vi "参数.vi"() -> ()   [LabVIEW 2018]
panel:
  in  "变频快速变化量":sgl caption="N" format="%.2f"
  in  "变频慢速变化量":sgl caption="N" format="%.2f"
  in  "变频变化周期":sgl caption="N" format="%.2f"
  in  "变频初始频率":sgl caption="N" format="%.2f"
  out "信号":bool
  out "物料编号":string
  out "机台编号":string
  out "产线编号":string
  in  "选项卡控件":enum32{"出风口", "信号显示"}(tab)
  in  "1#选项卡控件":enum32{"拨钮左到右", "拨钮右到左", "拨钮下到上", "拨钮上到下"}(tab)
  in  "1#拨钮左右-系数+":sgl=10.0 caption="操作力系数+" format="%.2f"
  in  "1#拨钮左右-基准":sgl=10.0 caption="操作力基准" format="%.2f"
  in  "1#拨钮左右-上参考":sgl=10.0 caption="操作力上参考" format="%.2f"
  in  "1#拨钮左右-下参考":sgl=10.0 caption="操作力下参考" format="%.2f"
  in  "1#拨钮左右-终点":dbl=10.0 caption="操作力终点" format="%.2f"
  in  "1#拨钮左右-起点":dbl=10.0 caption="操作力起点" format="%.2f"
  in  "1#拨钮左右-锁起点":dbl=10.0 caption="锁止力起点" format="%.2f"
  in  "1#拨钮左右-锁终点":dbl=10.0 caption="锁止力终点" format="%.2f"
  in  "1#拨钮左右-锁系数+":sgl=10.0 caption="锁止力系数+" format="%.2f"
  in  "1#拨钮左右-锁系数x":sgl=10.0 caption="锁止力系数x" format="%.2f"
  in  "1#拨钮左右-锁上限":sgl=10.0 caption="锁止力上限" format="%.2f"
  in  "1#拨钮左右-锁下限":sgl=10.0 caption="锁止力下限" format="%.2f"
  in  "1#拨钮左右-系数x":sgl=10.0 caption="操作力系数x" format="%.2f"
  in  "1#拨钮左右-曲线点数":dbl=10.0 caption="曲线点数"
  in  "1#拨钮左右-上限":sgl=10.0 caption="操作力上限" format="%.2f"
  in  "1#拨钮左右-下限":sgl=10.0 caption="操作力下限" format="%.2f"
  in  "1#拨钮左右-Y轴上限":dbl=10.0 caption="Y轴上限" format="%.1f"
  in  "1#拨钮左右-Y轴下限":dbl=10.0 caption="Y轴下限" format="%.1f"
  in  "1#拨钮右左-系数+":sgl=10.0 caption="操作力系数+" format="%.2f"
  in  "1#拨钮右左-基准":sgl=10.0 caption="操作力基准" format="%.2f"
  in  "1#拨钮右左上参考":sgl=10.0 caption="操作力上参考" format="%.2f"
  in  "1#拨钮右左-下参考":sgl=10.0 caption="操作力下参考" format="%.2f"
  in  "1#拨钮右左-终点":dbl=10.0 caption="操作力终点" format="%.2f"
  in  "1#拨钮右左-起点":dbl=10.0 caption="操作力起点" format="%.2f"
  in  "1#拨钮右左-锁起点":dbl=10.0 caption="锁止力起点" format="%.2f"
  in  "1#拨钮右左-锁终点":dbl=10.0 caption="锁止力终点" format="%.2f"
  in  "1#拨钮右左-锁系数+":sgl=10.0 caption="锁止力系数+" format="%.2f"
  in  "1#拨钮右左-锁系数x":sgl=10.0 caption="锁止力系数x" format="%.2f"
  in  "1#拨钮右左-锁上限":sgl=10.0 caption="锁止力上限" format="%.2f"
  in  "1#拨钮右左-锁下限":sgl=10.0 caption="锁止力下限" format="%.2f"
  in  "1#拨钮右左-系数x":sgl=10.0 caption="操作力系数x" format="%.2f"
  in  "1#拨钮右左-曲线点数":dbl=10.0 caption="曲线点数"
  in  "1#拨钮右左-上限":sgl=10.0 caption="操作力上限" format="%.2f"
  in  "1#拨钮右左-下限":sgl=10.0 caption="操作力下限" format="%.2f"
  in  "1#拨钮右左-Y轴上限":dbl=10.0 caption="Y轴上限" format="%.1f"
  in  "1#拨钮右左-Y轴下限":dbl=10.0 caption="Y轴下限" format="%.1f"
  in  "1#拨钮下上-系数+":sgl=10.0 caption="操作力系数+" format="%.2f"
  in  "1#拨钮下上-基准":sgl=10.0 caption="操作力基准" format="%.2f"
  in  "1#拨钮下上-上参考":sgl=10.0 caption="操作力上参考" format="%.2f"
  in  "1#拨钮下上-下参考":sgl=10.0 caption="操作力下参考" format="%.2f"
  in  "1#拨钮下上-终点":dbl=10.0 caption="操作力终点" format="%.2f"
  in  "1#拨钮下上-起点":dbl=10.0 caption="操作力起点" format="%.2f"
  in  "1#拨钮下上-系数x":sgl=10.0 caption="操作力系数x" format="%.2f"
  in  "1#拨钮下上-曲线点数":dbl=10.0 caption="曲线点数"
  in  "1#拨钮下上-上限":sgl=10.0 caption="操作力上限" format="%.2f"
  in  "1#拨钮下上-下限":sgl=10.0 caption="操作力下限" format="%.2f"
  in  "1#拨钮下上-Y轴上限":dbl=10.0 caption="Y轴上限" format="%.1f"
  in  "1#拨钮下上-Y轴下限":dbl=10.0 caption="Y轴下限" format="%.1f"
  in  "1#拨钮上下-系数+":sgl=10.0 caption="操作力系数+" format="%.2f"
  in  "1#拨钮上下-基准":sgl=10.0 caption="操作力基准" format="%.2f"
  in  "1#拨钮上下-上参考":sgl=10.0 caption="操作力上参考" format="%.2f"
  in  "1#拨钮上下-下参考":sgl=10.0 caption="操作力下参考" format="%.2f"
  in  "1#拨钮上下-终点":dbl=10.0 caption="操作力终点" format="%.2f"
  in  "1#拨钮上下-起点":dbl=10.0 caption="操作力起点" format="%.2f"
  in  "1#拨钮上下-系数x":sgl=10.0 caption="操作力系数x" format="%.2f"
  in  "1#拨钮上下-曲线点数":dbl=10.0 caption="曲线点数"
  in  "1#拨钮上下-上限":sgl=10.0 caption="操作力上限" format="%.2f"
  in  "1#拨钮上下-下限":sgl=10.0 caption="操作力下限" format="%.2f"
  in  "1#拨钮上下-Y轴上限":dbl=10.0 caption="Y轴上限" format="%.1f"
  in  "1#拨钮上下-Y轴下限":dbl=10.0 caption="Y轴下限" format="%.1f"
  out "检测序号":u16 format="%05d"
  out "力":sgl[](array[numeric]) format="%.4f"
  out "PLC结果":T1
  out "检测步骤":T2
  out "PLC状态":T3
  in  "LOG":bool
  in  "伺服速度":sgl caption="N" format="%.1f"
  in  "气压稳定时间":sgl caption="N" format="%.1f"
  in  "LED电流下限":sgl caption="N" format="%.2f"
  in  "LED电流上限":sgl caption="N" format="%.2f"
  in  "风门开电压下限":sgl caption="N" format="%.2f"
  in  "风门开电压上限":sgl caption="N" format="%.2f"
  in  "风门闭电压下限":sgl caption="N" format="%.2f"
  in  "风门闭电压上限":sgl caption="N" format="%.2f"
  in  "压力下限":sgl caption="N" format="%.1f"
  in  "压力上限":sgl caption="N" format="%.1f"
  in  "泄漏量上限":sgl caption="N" format="%.2f"
  out "有值改变":bool
  in  "停止":bool
  in  "轮盘预压力":sgl caption="N" format="%.1f"
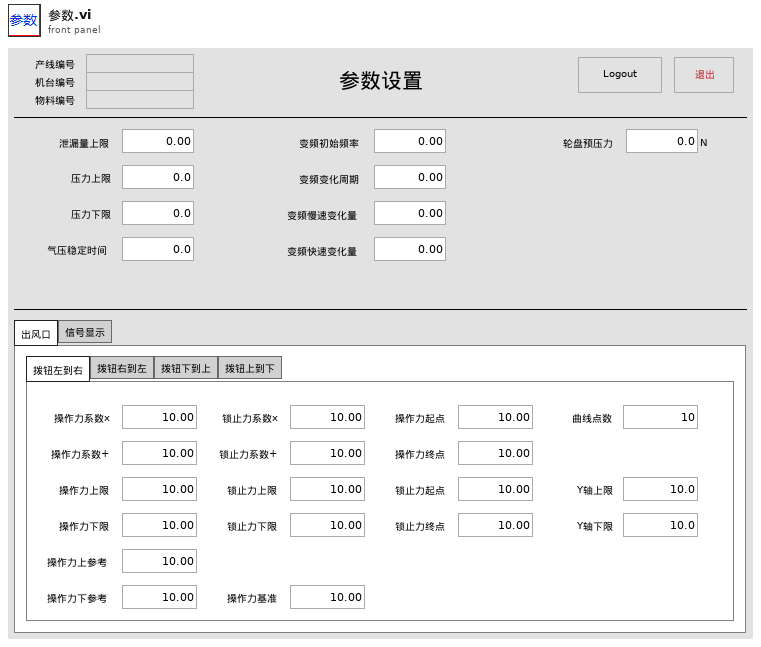
[diagram p1: front panel]
types:
  T1 = cluster{"1#泄漏量":bool, "1#风门闭电压":bool, "1#风门开电压":bool, "1#LED电压":bool, "1#LED电流":bool, "外观结果":bool, "2#泄漏量":bool, "2#风门闭电压":bool, "2#风门开电压":bool, "2#LED电压":bool, "2#LED电流":bool, "3#泄漏量":bool, "3#风门闭电压":bool, "3#风门开电压":bool, "3#LED电压":bool, "3#LED电流":bool}
  T2 = cluster{"泄漏量":bool, "风门开闭电检":bool, "LED电检":bool, "外观检测":bool, "1#轮盘关开":bool, "1#轮盘关开锁":bool, "1#轮盘开关":bool, "1#轮盘开关锁":bool, "1#拨钮左右":bool, "1#拨钮右左":bool, "1#拨钮上下":bool, "1#拨钮下上":bool, "2#轮盘关开":bool, "2#轮盘关开锁":bool, "2#轮盘开关":bool, "2#轮盘开关锁":bool, "2#拨钮左右":bool, "2#拨钮右左":bool, "2#拨钮上下":bool, "2#拨钮下上":bool, "3#轮盘关开":bool, "3#轮盘关开锁":bool, "3#轮盘开关":bool, "3#轮盘开关锁":bool, "3#拨钮左右":bool, "3#拨钮右左":bool, "3#拨钮上下":bool, "3#拨钮下上":bool}
  T3 = cluster{"PLC就绪":bool, "ROBOT就绪":bool, "空动作":bool, "检测NG":bool, "检测结束":bool, "检测开始":bool, "初始化脉冲":bool, "1#检测NG":bool, "2#检测NG":bool, "3#检测NG":bool}
  T4 = enum8{"Enabled", "Disabled", "Disabled and Grayed Out"}
  T5 = cluster{"轮盘预压力":sgl, "泄漏量上限":sgl, "压力上限":sgl, "压力下限":sgl, "风门闭电压上限":sgl, "风门闭电压下限":sgl, "风门开电压上限":sgl, "风门开电压下限":sgl, "LED电流上限":sgl, "LED电流下限":sgl, "气压稳定时间":sgl, "伺服速度":sgl, "INV初始频率":sgl, "INV变化周期":sgl, "INV慢速变化量":sgl, "INV快速变化量":sgl}
  T6 = cluster{"选择":enum16{"Fx", "Fy", "Fz", "Mx", "My", "Mz"}, "系数x":sgl, "系数+":sgl, "上限":sgl, "下限":sgl, "Ymax":dbl, "Ymin":dbl, "点数":dbl, "锁系数x":sgl, "锁上限":sgl, "锁下限":sgl, "锁系数+":sgl, "起点":dbl, "终点":dbl, "锁起点":dbl, "锁终点":dbl, "上参考":sgl, "下参考":sgl, "基准":sgl}
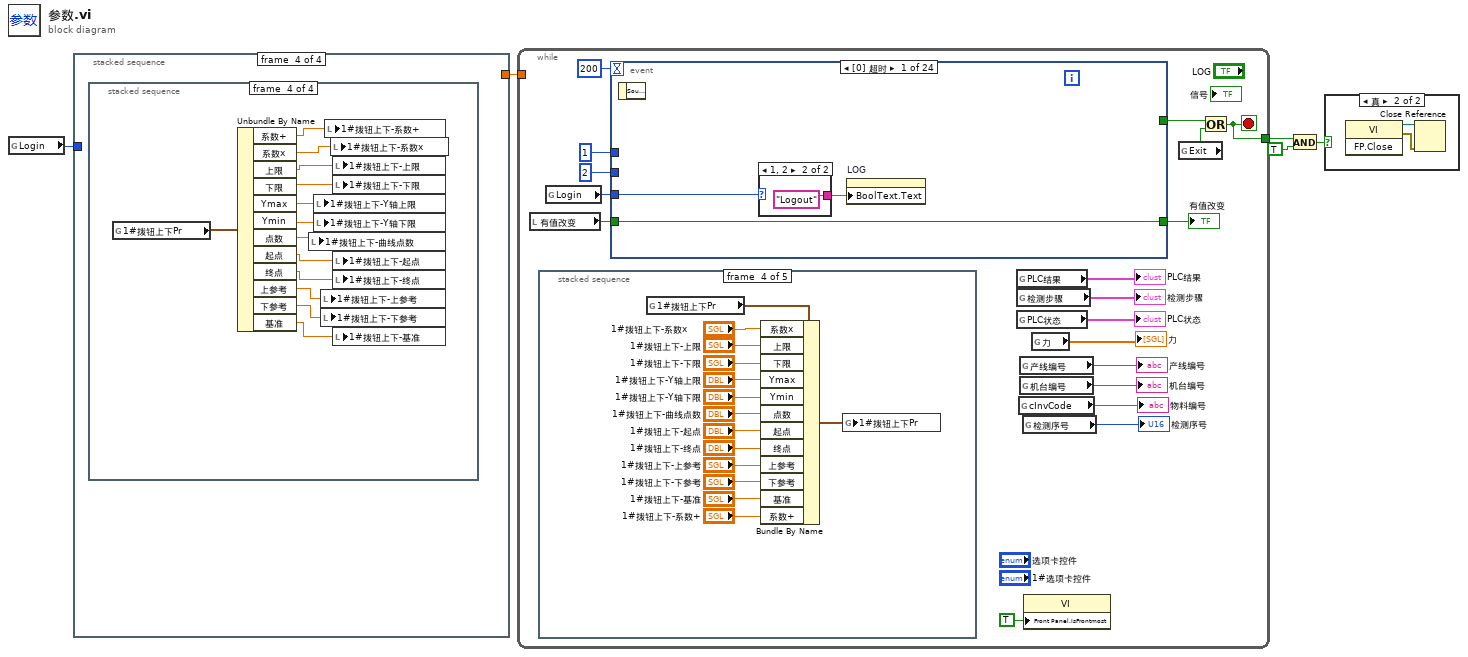
[diagram p0: block diagram]
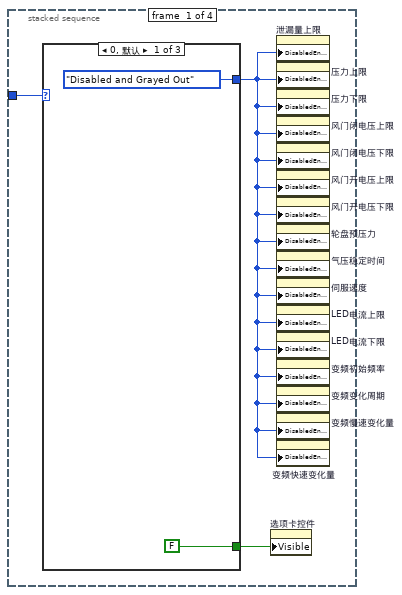
[diagram p2: hidden frame]
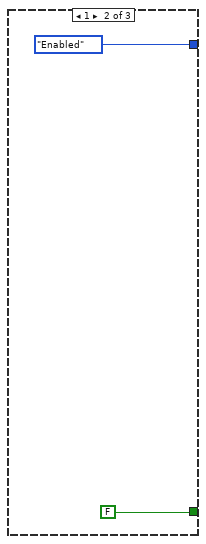
[diagram p3: hidden frame]
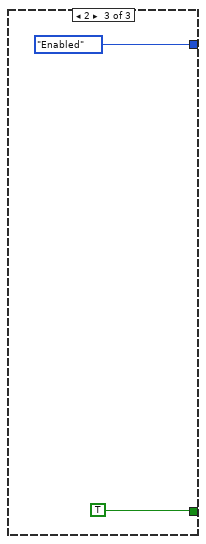
[diagram p4: hidden frame]
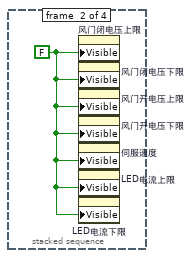
[diagram p5: hidden frame]
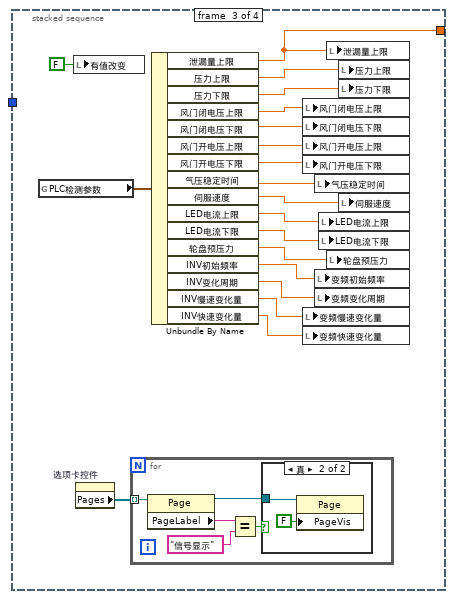
[diagram p6: hidden frame]
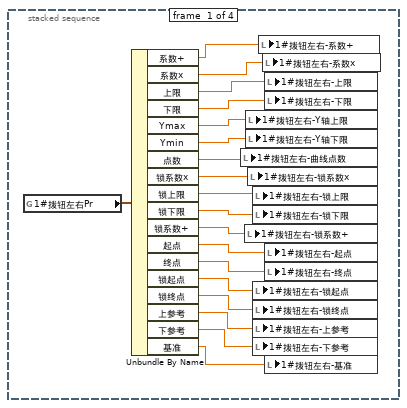
[diagram p8: hidden frame]
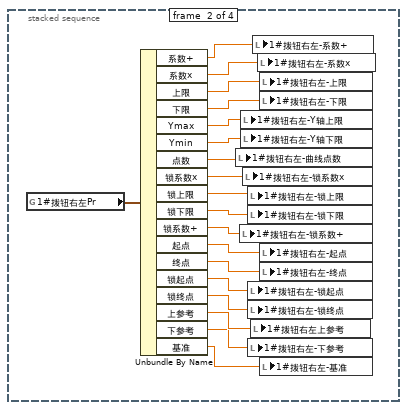
[diagram p9: hidden frame]
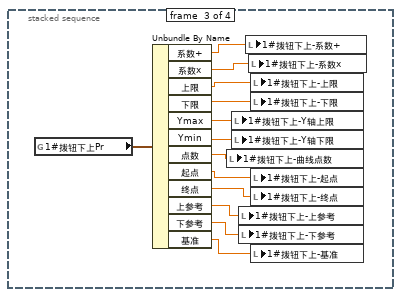
[diagram p10: hidden frame]
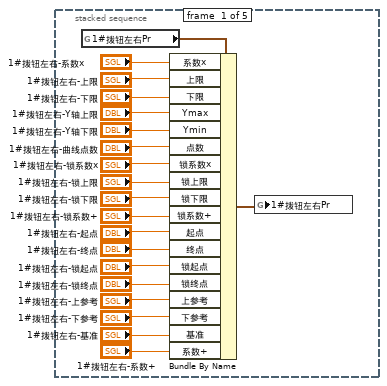
[diagram p12: hidden frame]
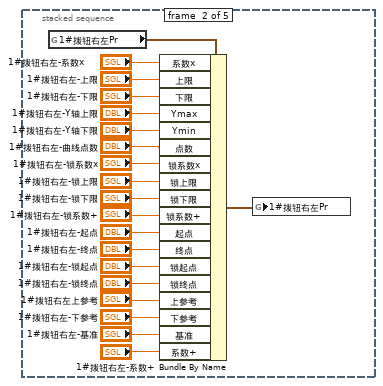
[diagram p13: hidden frame]
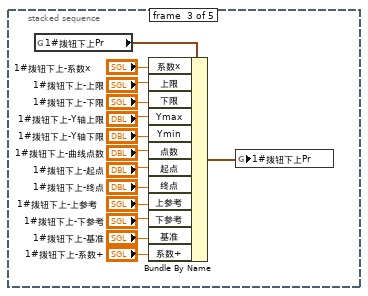
[diagram p14: hidden frame]
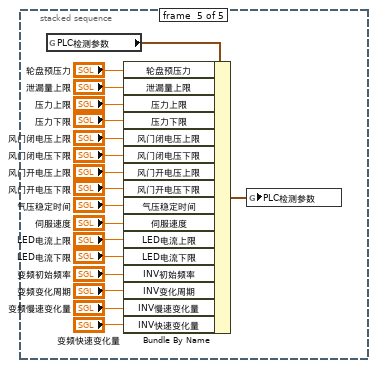
[diagram p15: hidden frame]
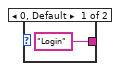
[diagram p16: hidden frame]
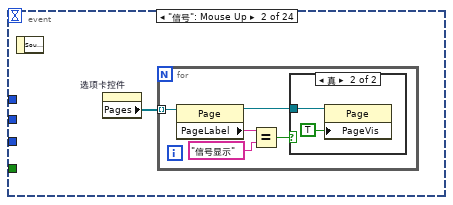
[diagram p17: hidden frame]
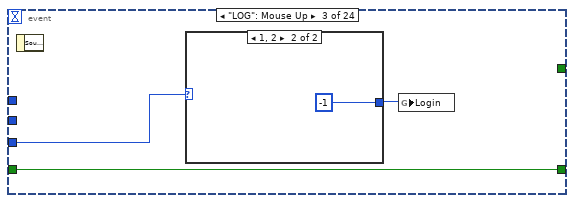
[diagram p19: hidden frame]
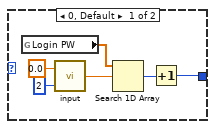
[diagram p20: hidden frame]
diagram:
  n1 = global read "全局 1.vi" "Login"() -> (w2:i32)
  n2 = stacked-sequence {
    tunnel: w2 -> [w8 _ _ _]
    tunnel: [_ _ w20 _] -> w1
    frame #0 {
      n3 = case shown="0, 默认" w8 {
        tunnel: [T4."Disabled and Grayed Out" ("禁用") T4."Enabled" ("禁用") T4."Enabled" ("禁用")] -> w6
        tunnel: [FALSE ("可见") FALSE ("可见") TRUE ("可见")] -> w7
        frame 0, Default {
        }
        frame 1 {
        }
        frame 2 {
        }
      }
      n4 = property on="选项卡控件" class="TabCtl (严格)"("Visible"=w7) -> ()  [unwired: 2 in, 2 out]
      n5 = property on="泄漏量上限" class="DigNum (严格)"("DisabledEnum"=w6) -> ()  [unwired: 2 in, 2 out]
      n6 = property on="压力上限" class="DigNum (严格)"("DisabledEnum"=w6) -> ()  [unwired: 2 in, 2 out]
      n7 = property on="压力下限" class="DigNum (严格)"("DisabledEnum"=w6) -> ()  [unwired: 2 in, 2 out]
      n8 = property on="风门闭电压上限" class="DigNum (严格)"("DisabledEnum"=w6) -> ()  [unwired: 2 in, 2 out]
      n9 = property on="风门闭电压下限" class="DigNum (严格)"("DisabledEnum"=w6) -> ()  [unwired: 2 in, 2 out]
      n10 = property on="风门开电压上限" class="DigNum (严格)"("DisabledEnum"=w6) -> ()  [unwired: 2 in, 2 out]
      n11 = property on="风门开电压下限" class="DigNum (严格)"("DisabledEnum"=w6) -> ()  [unwired: 2 in, 2 out]
      n12 = property on="轮盘预压力" class="DigNum (严格)"("DisabledEnum"=w6) -> ()  [unwired: 2 in, 2 out]
      n13 = property on="气压稳定时间" class="DigNum (严格)"("DisabledEnum"=w6) -> ()  [unwired: 2 in, 2 out]
      n14 = property on="伺服速度" class="DigNum (严格)"("DisabledEnum"=w6) -> ()  [unwired: 2 in, 2 out]
      n15 = property on="LED电流上限" class="DigNum (严格)"("DisabledEnum"=w6) -> ()  [unwired: 2 in, 2 out]
      n16 = property on="LED电流下限" class="DigNum (严格)"("DisabledEnum"=w6) -> ()  [unwired: 2 in, 2 out]
      n17 = property on="变频初始频率" class="DigNum (严格)"("DisabledEnum"=w6) -> ()  [unwired: 2 in, 2 out]
      n18 = property on="变频变化周期" class="DigNum (严格)"("DisabledEnum"=w6) -> ()  [unwired: 2 in, 2 out]
      n19 = property on="变频慢速变化量" class="DigNum (严格)"("DisabledEnum"=w6) -> ()  [unwired: 2 in, 2 out]
      n20 = property on="变频快速变化量" class="DigNum (严格)"("DisabledEnum"=w6) -> ()  [unwired: 2 in, 2 out]
    }
    frame #1 {
      w15 = FALSE ("可见")
      n21 = property on="风门闭电压上限" class="DigNum (严格)"("Visible"=w15) -> ()  [unwired: 2 in, 2 out]
      n22 = property on="风门闭电压下限" class="DigNum (严格)"("Visible"=w15) -> ()  [unwired: 2 in, 2 out]
      n23 = property on="风门开电压上限" class="DigNum (严格)"("Visible"=w15) -> ()  [unwired: 2 in, 2 out]
      n24 = property on="风门开电压下限" class="DigNum (严格)"("Visible"=w15) -> ()  [unwired: 2 in, 2 out]
      n25 = property on="伺服速度" class="DigNum (严格)"("Visible"=w15) -> ()  [unwired: 2 in, 2 out]
      n26 = property on="LED电流上限" class="DigNum (严格)"("Visible"=w15) -> ()  [unwired: 2 in, 2 out]
      n27 = property on="LED电流下限" class="DigNum (严格)"("Visible"=w15) -> ()  [unwired: 2 in, 2 out]
    }
    frame #2 {
      n28 = global read "全局 1.vi" "PLC检测参数"() -> (w24:T5)
      n29 = local write "有值改变"(FALSE ("有值改变")) -> ()
      n30 = property on="选项卡控件" class="TabCtl (严格)"() -> ("Pages"=w21:refnum<vi>[])  [unwired: 2 in, 2 out]
      n31 = for {
        tunnel: w21 -> [w36] mode=indexing
        n32 = property class="Page"(reference=w36) -> (reference out=w35:refnum<vi>, "PageLabel"=w39:string)  [unwired: 1 in, 1 out]
        n33 = Equal?(x=w39, y="信号显示") -> (x = y?=w37:bool)
        n34 = case shown="真" w37 {
          tunnel: w35 -> [_ w40]
          frame False {
          }
          frame True {
            n35 = property class="Page"(reference=w40, "PageVis"=FALSE ("选项卡可见")) -> ()  [unwired: 1 in, 2 out]
          }
        }
      }
      n36 = Unbundle By Name(w24) -> ("泄漏量上限"=w20:sgl, "压力上限"=w34:sgl, "压力下限"=w33:sgl, "风门闭电压上限"=w32:sgl, "风门闭电压下限"=w31:sgl, "风门开电压上限"=w30:sgl, "风门开电压下限"=w29:sgl, "气压稳定时间"=w28:sgl, "伺服速度"=w27:sgl, "LED电流上限"=w26:sgl, "LED电流下限"=w25:sgl, "轮盘预压力"=w22:sgl, "INV初始频率"=w16:sgl, "INV变化周期"=w17:sgl, "INV慢速变化量"=w18:sgl, "INV快速变化量"=w19:sgl)
      n37 = local write "风门闭电压上限"(w32) -> ()
      n38 = local write "风门闭电压下限"(w31) -> ()
      n39 = local write "风门开电压上限"(w30) -> ()
      n40 = local write "风门开电压下限"(w29) -> ()
      n41 = local write "变频慢速变化量"(w18) -> ()
      n42 = local write "变频快速变化量"(w19) -> ()
      n43 = local write "气压稳定时间"(w28) -> ()
      n44 = local write "变频初始频率"(w16) -> ()
      n45 = local write "变频变化周期"(w17) -> ()
      n46 = local write "LED电流上限"(w26) -> ()
      n47 = local write "LED电流下限"(w25) -> ()
      n48 = local write "泄漏量上限"(w20) -> ()
      n49 = local write "轮盘预压力"(w22) -> ()
      n50 = local write "压力上限"(w34) -> ()
      n51 = local write "压力下限"(w33) -> ()
      n52 = local write "伺服速度"(w27) -> ()
    }
    frame #3 {
      n53 = stacked-sequence {
        frame #0 {
          n54 = global read "全局F参数.vi" "1#拨钮左右Pr"() -> (w60:T6)
          n55 = Unbundle By Name(w60) -> ("系数+"=w42:sgl, "系数x"=w59:sgl, "上限"=w57:sgl, "下限"=w56:sgl, "Ymax"=w55:dbl, "Ymin"=w54:dbl, "点数"=w58:dbl, "锁系数x"=w51:sgl, "锁上限"=w53:sgl, "锁下限"=w52:sgl, "锁系数+"=w50:sgl, "起点"=w49:dbl, "终点"=w48:dbl, "锁起点"=w47:dbl, "锁终点"=w46:dbl, "上参考"=w45:sgl, "下参考"=w44:sgl, "基准"=w43:sgl)
          n56 = local write "1#拨钮左右-曲线点数"(w58) -> ()
          n57 = local write "1#拨钮左右-锁系数+"(w50) -> ()
          n58 = local write "1#拨钮左右-Y轴上限"(w55) -> ()
          n59 = local write "1#拨钮左右-Y轴下限"(w54) -> ()
          n60 = local write "1#拨钮左右-锁系数x"(w51) -> ()
          n61 = local write "1#拨钮左右-锁上限"(w53) -> ()
          n62 = local write "1#拨钮左右-锁下限"(w52) -> ()
          n63 = local write "1#拨钮左右-锁起点"(w47) -> ()
          n64 = local write "1#拨钮左右-锁终点"(w46) -> ()
          n65 = local write "1#拨钮左右-上参考"(w45) -> ()
          n66 = local write "1#拨钮左右-下参考"(w44) -> ()
          n67 = local write "1#拨钮左右-系数+"(w42) -> ()
          n68 = local write "1#拨钮左右-系数x"(w59) -> ()
          n69 = local write "1#拨钮左右-上限"(w57) -> ()
          n70 = local write "1#拨钮左右-下限"(w56) -> ()
          n71 = local write "1#拨钮左右-起点"(w49) -> ()
          n72 = local write "1#拨钮左右-终点"(w48) -> ()
          n73 = local write "1#拨钮左右-基准"(w43) -> ()
        }
        frame #1 {
          n74 = global read "全局F参数.vi" "1#拨钮右左Pr"() -> (w79:T6)
          n75 = Unbundle By Name(w79) -> ("系数+"=w61:sgl, "系数x"=w78:sgl, "上限"=w76:sgl, "下限"=w75:sgl, "Ymax"=w74:dbl, "Ymin"=w73:dbl, "点数"=w77:dbl, "锁系数x"=w72:sgl, "锁上限"=w71:sgl, "锁下限"=w70:sgl, "锁系数+"=w69:sgl, "起点"=w68:dbl, "终点"=w67:dbl, "锁起点"=w66:dbl, "锁终点"=w65:dbl, "上参考"=w64:sgl, "下参考"=w63:sgl, "基准"=w62:sgl)
          n76 = local write "1#拨钮右左-曲线点数"(w77) -> ()
          n77 = local write "1#拨钮右左-锁系数+"(w69) -> ()
          n78 = local write "1#拨钮右左-Y轴上限"(w74) -> ()
          n79 = local write "1#拨钮右左-Y轴下限"(w73) -> ()
          n80 = local write "1#拨钮右左-锁系数x"(w72) -> ()
          n81 = local write "1#拨钮右左-锁上限"(w71) -> ()
          n82 = local write "1#拨钮右左-锁下限"(w70) -> ()
          n83 = local write "1#拨钮右左-锁起点"(w66) -> ()
          n84 = local write "1#拨钮右左-锁终点"(w65) -> ()
          n85 = local write "1#拨钮右左-下参考"(w63) -> ()
          n86 = local write "1#拨钮右左上参考"(w64) -> ()
          n87 = local write "1#拨钮右左-系数+"(w61) -> ()
          n88 = local write "1#拨钮右左-系数x"(w78) -> ()
          n89 = local write "1#拨钮右左-上限"(w76) -> ()
          n90 = local write "1#拨钮右左-下限"(w75) -> ()
          n91 = local write "1#拨钮右左-起点"(w68) -> ()
          n92 = local write "1#拨钮右左-终点"(w67) -> ()
          n93 = local write "1#拨钮右左-基准"(w62) -> ()
        }
        frame #2 {
          n94 = global read "全局F参数.vi" "1#拨钮下上Pr"() -> (w92:T6)
          n95 = Unbundle By Name(w92) -> ("系数+"=w80:sgl, "系数x"=w91:sgl, "上限"=w89:sgl, "下限"=w88:sgl, "Ymax"=w87:dbl, "Ymin"=w86:dbl, "点数"=w90:dbl, "起点"=w85:dbl, "终点"=w84:dbl, "上参考"=w83:sgl, "下参考"=w82:sgl, "基准"=w81:sgl)
          n96 = local write "1#拨钮下上-曲线点数"(w90) -> ()
          n97 = local write "1#拨钮下上-Y轴上限"(w87) -> ()
          n98 = local write "1#拨钮下上-Y轴下限"(w86) -> ()
          n99 = local write "1#拨钮下上-上参考"(w83) -> ()
          n100 = local write "1#拨钮下上-下参考"(w82) -> ()
          n101 = local write "1#拨钮下上-系数+"(w80) -> ()
          n102 = local write "1#拨钮下上-系数x"(w91) -> ()
          n103 = local write "1#拨钮下上-上限"(w89) -> ()
          n104 = local write "1#拨钮下上-下限"(w88) -> ()
          n105 = local write "1#拨钮下上-起点"(w85) -> ()
          n106 = local write "1#拨钮下上-终点"(w84) -> ()
          n107 = local write "1#拨钮下上-基准"(w81) -> ()
        }
        frame #3 {
          n108 = global read "全局F参数.vi" "1#拨钮上下Pr"() -> (w105:T6)
          n109 = Unbundle By Name(w105) -> ("系数+"=w93:sgl, "系数x"=w104:sgl, "上限"=w102:sgl, "下限"=w101:sgl, "Ymax"=w100:dbl, "Ymin"=w99:dbl, "点数"=w103:dbl, "起点"=w97:dbl, "终点"=w98:dbl, "上参考"=w96:sgl, "下参考"=w95:sgl, "基准"=w94:sgl)
          n110 = local write "1#拨钮上下-曲线点数"(w103) -> ()
          n111 = local write "1#拨钮上下-Y轴上限"(w100) -> ()
          n112 = local write "1#拨钮上下-Y轴下限"(w99) -> ()
          n113 = local write "1#拨钮上下-上参考"(w96) -> ()
          n114 = local write "1#拨钮上下-下参考"(w95) -> ()
          n115 = local write "1#拨钮上下-系数+"(w93) -> ()
          n116 = local write "1#拨钮上下-系数x"(w104) -> ()
          n117 = local write "1#拨钮上下-上限"(w102) -> ()
          n118 = local write "1#拨钮上下-下限"(w101) -> ()
          n119 = local write "1#拨钮上下-起点"(w97) -> ()
          n120 = local write "1#拨钮上下-终点"(w98) -> ()
          n121 = local write "1#拨钮上下-基准"(w94) -> ()
        }
      }
    }
  }
  n122 = while {
    tunnel: [w120] -> w4
    tunnel: w1 -> [_]
    stop <- w120 stop-if-true
    n123 = local read "有值改变"() -> (w114:bool)
    n124 = stacked-sequence {
      frame #0 {
        n125 = global read "全局F参数.vi" "1#拨钮左右Pr"() -> (w143:T6)
        n126 = Bundle By Name(cluster=w143, "系数x"="1#拨钮左右-系数x", "上限"="1#拨钮左右-上限", "下限"="1#拨钮左右-下限", "Ymax"="1#拨钮左右-Y轴上限", "Ymin"="1#拨钮左右-Y轴下限", "点数"="1#拨钮左右-曲线点数", "锁系数x"="1#拨钮左右-锁系数x", "锁上限"="1#拨钮左右-锁上限", "锁下限"="1#拨钮左右-锁下限", "锁系数+"="1#拨钮左右-锁系数+", "起点"="1#拨钮左右-起点", "终点"="1#拨钮左右-终点", "锁起点"="1#拨钮左右-锁起点", "锁终点"="1#拨钮左右-锁终点", "上参考"="1#拨钮左右-上参考", "下参考"="1#拨钮左右-下参考", "基准"="1#拨钮左右-基准", "系数+"="1#拨钮左右-系数+") -> (w136:T6)
        n127 = global write "全局F参数.vi" "1#拨钮左右Pr"(w136) -> ()
      }
      frame #1 {
        n128 = global read "全局F参数.vi" "1#拨钮右左Pr"() -> (w163:T6)
        n129 = Bundle By Name(cluster=w163, "系数x"="1#拨钮右左-系数x", "上限"="1#拨钮右左-上限", "下限"="1#拨钮右左-下限", "Ymax"="1#拨钮右左-Y轴上限", "Ymin"="1#拨钮右左-Y轴下限", "点数"="1#拨钮右左-曲线点数", "锁系数x"="1#拨钮右左-锁系数x", "锁上限"="1#拨钮右左-锁上限", "锁下限"="1#拨钮右左-锁下限", "锁系数+"="1#拨钮右左-锁系数+", "起点"="1#拨钮右左-起点", "终点"="1#拨钮右左-终点", "锁起点"="1#拨钮右左-锁起点", "锁终点"="1#拨钮右左-锁终点", "上参考"="1#拨钮右左上参考", "下参考"="1#拨钮右左-下参考", "基准"="1#拨钮右左-基准", "系数+"="1#拨钮右左-系数+") -> (w162:T6)
        n130 = global write "全局F参数.vi" "1#拨钮右左Pr"(w162) -> ()
      }
      frame #2 {
        n131 = global read "全局F参数.vi" "1#拨钮下上Pr"() -> (w177:T6)
        n132 = Bundle By Name(cluster=w177, "系数x"="1#拨钮下上-系数x", "上限"="1#拨钮下上-上限", "下限"="1#拨钮下上-下限", "Ymax"="1#拨钮下上-Y轴上限", "Ymin"="1#拨钮下上-Y轴下限", "点数"="1#拨钮下上-曲线点数", "起点"="1#拨钮下上-起点", "终点"="1#拨钮下上-终点", "上参考"="1#拨钮下上-上参考", "下参考"="1#拨钮下上-下参考", "基准"="1#拨钮下上-基准", "系数+"="1#拨钮下上-系数+") -> (w176:T6)
        n133 = global write "全局F参数.vi" "1#拨钮下上Pr"(w176) -> ()
      }
      frame #3 {
        n134 = global read "全局F参数.vi" "1#拨钮上下Pr"() -> (w191:T6)
        n135 = Bundle By Name(cluster=w191, "系数x"="1#拨钮上下-系数x", "上限"="1#拨钮上下-上限", "下限"="1#拨钮上下-下限", "Ymax"="1#拨钮上下-Y轴上限", "Ymin"="1#拨钮上下-Y轴下限", "点数"="1#拨钮上下-曲线点数", "起点"="1#拨钮上下-起点", "终点"="1#拨钮上下-终点", "上参考"="1#拨钮上下-上参考", "下参考"="1#拨钮上下-下参考", "基准"="1#拨钮上下-基准", "系数+"="1#拨钮上下-系数+") -> (w190:T6)
        n136 = global write "全局F参数.vi" "1#拨钮上下Pr"(w190) -> ()
      }
      frame #4 {
        n137 = global read "全局 1.vi" "PLC检测参数"() -> (w196:T5)
        n138 = Bundle By Name(cluster=w196, "轮盘预压力"="轮盘预压力", "泄漏量上限"="泄漏量上限", "压力上限"="压力上限", "压力下限"="压力下限", "风门闭电压上限"="风门闭电压上限", "风门闭电压下限"="风门闭电压下限", "风门开电压上限"="风门开电压上限", "风门开电压下限"="风门开电压下限", "气压稳定时间"="气压稳定时间", "伺服速度"="伺服速度", "LED电流上限"="LED电流上限", "LED电流下限"="LED电流下限", "INV初始频率"="变频初始频率", "INV变化周期"="变频变化周期", "INV慢速变化量"="变频慢速变化量", "INV快速变化量"="变频快速变化量") -> (w209:T5)
        n139 = global write "全局 1.vi" "PLC检测参数"(w209) -> ()
      }
    }
    n140 = global read "全局 1.vi" "Login"() -> (w115:i32)
    n141 = event shown="[0] 超时" {
      selector: _ -> [_ _ _ _ _ _ _ _ _ _ _ _ _ _ _ _ _ _ _ _ _ _ _ _]
      dyn-events: _ -> [_ _ _ _ _ _ _ _ _ _ _ _ _ _ _ _ _ _ _ _ _ _ _ _]
      timeout: 200 -> [_ _ _ _ _ _ _ _ _ _ _ _ _ _ _ _ _ _ _ _ _ _ _ _]
      tunnel: [_ _ _ "停止" _ _ _ _ _ _ _ _ _ _ _ _ _ _ _ _ _ _ _ _] -> w119
      tunnel: 1 -> [_ _ _ _ w241 _ _ _ _ _ _ _ _ _ _ _ _ _ _ _ _ w369 w376 _]
      tunnel: 2 -> [_ _ _ _ _ w254 w263 w270 w277 w284 w293 w300 w307 w314 w321 w328 w335 w342 w349 w356 w363 _ _ _]
      tunnel: [w210 _ w224 w233 w240 w253 w265 w272 w279 w286 w292 w299 w306 w313 w320 w327 w334 w341 w348 w355 w362 w370 w377 w384] -> w116
      tunnel: w115 -> [w212 _ w225 _ _ _ _ _ _ _ _ _ _ _ _ _ _ _ _ _ _ _ _ _]
      tunnel: w114 -> [w210 _ w224 w233 w239 w252 _ _ _ _ _ _ _ _ _ _ _ _ _ _ _ _ _ _]
      event Timeout {
        n142 = event-data() -> ()  [unwired: 1 in, 1 out]
        n143 = case shown="1, 2" w212 {
          tunnel: ["Login" "Logout"] -> w211
          frame 0, Default {
          }
          frame 1, 2 {
          }
        }
        n144 = property on="LOG" class="Bool"("BoolText.Text"=w211) -> ()  [unwired: 2 in, 2 out]
      }
      event "信号": Mouse Up {
        n145 = event-data() -> ()  [unwired: 1 in, 1 out]
        n146 = property on="选项卡控件" class="TabCtl (严格)"() -> ("Pages"=w215:refnum<vi>[])  [unwired: 2 in, 2 out]
        n147 = for {
          tunnel: w215 -> [w217] mode=indexing
          n148 = property class="Page"(reference=w217) -> (reference out=w216:refnum<vi>, "PageLabel"=w220:string)  [unwired: 1 in, 1 out]
          n149 = Equal?(x=w220, y="信号显示") -> (x = y?=w218:bool)
          n150 = case shown="真" w218 {
            tunnel: w216 -> [_ w221]
            frame False {
            }
            frame True {
              n151 = property class="Page"(reference=w221, "PageVis"=TRUE ("选项卡可见")) -> ()  [unwired: 1 in, 2 out]
            }
          }
        }
      }
      event "LOG": Mouse Up {
        n152 = event-data() -> ()  [unwired: 1 in, 1 out]
        n153 = case shown="1, 2" w225 {
          tunnel: [w226 -1 ("index of element")] -> w223
          frame 0, Default {
            n154 = global read "全局 1.vi" "Login PW"() -> (w229:dbl[])
            n155 = call "input.vi"("位数(2)"=2, "in"=0.0) -> ("out"=w228:dbl)  [unwired: 1 out]
            n156 = Search 1D Array(1D array=w229, element=w228) -> (index of element=w227:i32)  [unwired: 1 in]
            n157 = Increment(x=w227) -> (x+1=w226:i32)
          }
          frame 1, 2 {
          }
        }
        n158 = global write "全局 1.vi" "Login"(w223) -> ()
      }
      event "停止": Value Change {
        n159 = event-data() -> ()  [unwired: 1 in, 1 out]
        n160 = global read "全局 1.vi" "ini文件"() -> (w234:path)
        n161 = case shown="真" w233 {
          tunnel: w234 -> [_ w236]
          frame False {
          }
          frame True {
            n162 = call "WriteIni.vi"("configuration file path"=w236) -> ()  [unwired: 1 in]
            n163 = call "WriteForceIni1#.vi"("configuration file path"=w236) -> ()  [unwired: 1 in]
          }
        }
      }
      event "压力上限", "压力下限", "气压稳定时间", "伺服速度", "轮盘预压力", "变频变化周期": Mouse Up {
        n164 = event-data() -> ("CtlRef"=w237:refnum<vi>)  [unwired: 1 in]
        n165 = property class="DigNum (严格)"(reference=w237) -> ("DisabledEnum"=w238:T4)  [unwired: 1 in, 2 out]
        n166 = case shown="\"Enabled\"" w238 {
          tunnel: w237 -> [w248 _]
          tunnel: w241 -> [w246 _]
          tunnel: [w245 w249] -> w240
          tunnel: w239 -> [_ w249]
          frame "Enabled" {
            n167 = property class="DigNum (严格)"(reference=w248) -> (reference out=w244:refnum<vi>, error out=w243:errorcluster, "Value"=w247:sgl)  [unwired: 1 in]
            n168 = call "input.vi"("位数(2)"=w246, "in"=w247) -> ("out"=w242:dbl, "值改变?"=w245:bool)
            n169 = property class="DigNum (严格)"(reference=w244, error in=w243, "Value"=w242) -> ()  [unwired: 2 out]
          }
          frame "Disabled", Default {
          }
        }
      }
      event "风门闭电压上限", "风门闭电压下限", "风门开电压上限", "风门开电压下限", "LED电流上限", "LED电流下限", "泄漏量上限", "变频初始频率", "变频慢速变化量", "变频快速变化量": Mouse Up {
        n170 = event-data() -> ("CtlRef"=w250:refnum<vi>)  [unwired: 1 in]
        n171 = property class="DigNum (严格)"(reference=w250) -> ("DisabledEnum"=w251:T4)  [unwired: 1 in, 2 out]
        n172 = case shown="\"Enabled\"" w251 {
          tunnel: w250 -> [w261 _]
          tunnel: w254 -> [w259 _]
          tunnel: [w258 w262] -> w253
          tunnel: w252 -> [_ w262]
          frame "Enabled" {
            n173 = property class="DigNum (严格)"(reference=w261) -> (reference out=w257:refnum<vi>, error out=w256:errorcluster, "Value"=w260:sgl)  [unwired: 1 in]
            n174 = call "input.vi"("位数(2)"=w259, "in"=w260) -> ("out"=w255:dbl, "值改变?"=w258:bool)
            n175 = property class="DigNum (严格)"(reference=w257, error in=w256, "Value"=w255) -> ()  [unwired: 2 out]
          }
          frame "Disabled", Default {
          }
        }
      }
      event "1#拨钮上下-系数x", "1#拨钮下上-系数x", "1#拨钮右左-系数x", "1#拨钮左右-系数x": Mouse Up {
        n176 = event-data() -> ("CtlRef"=w269:refnum<vi>)  [unwired: 1 in]
        n177 = property class="DigNum (严格)"(reference=w269) -> (reference out=w267:refnum<vi>, error out=w264:errorcluster, "Value"=w268:sgl)  [unwired: 1 in]
        n178 = call "input.vi"("位数(2)"=w263, "in"=w268) -> ("out"=w266:dbl, "值改变?"=w265:bool)
        n179 = property class="DigNum (严格)"(reference=w267, error in=w264, "Value"=w266) -> ()  [unwired: 2 out]
      }
      event "1#拨钮上下-系数+", "1#拨钮左右-系数+", "1#拨钮右左-系数+", "1#拨钮下上-系数+": Mouse Up {
        n180 = event-data() -> ("CtlRef"=w276:refnum<vi>)  [unwired: 1 in]
        n181 = property class="DigNum (严格)"(reference=w276) -> (reference out=w274:refnum<vi>, error out=w271:errorcluster, "Value"=w275:sgl)  [unwired: 1 in]
        n182 = call "input.vi"("位数(2)"=w270, "in"=w275) -> ("out"=w273:dbl, "值改变?"=w272:bool)
        n183 = property class="DigNum (严格)"(reference=w274, error in=w271, "Value"=w273) -> ()  [unwired: 2 out]
      }
      event "1#拨钮左右-锁系数x", "1#拨钮右左-锁系数x": Mouse Up {
        n184 = event-data() -> ("CtlRef"=w283:refnum<vi>)  [unwired: 1 in]
        n185 = property class="DigNum (严格)"(reference=w283) -> (reference out=w281:refnum<vi>, error out=w278:errorcluster, "Value"=w282:sgl)  [unwired: 1 in]
        n186 = call "input.vi"("位数(2)"=w277, "in"=w282) -> ("out"=w280:dbl, "值改变?"=w279:bool)
        n187 = property class="DigNum (严格)"(reference=w281, error in=w278, "Value"=w280) -> ()  [unwired: 2 out]
      }
      event "1#拨钮左右-锁系数+", "1#拨钮右左-锁系数+": Mouse Up {
        n188 = event-data() -> ("CtlRef"=w290:refnum<vi>)  [unwired: 1 in]
        n189 = property class="DigNum (严格)"(reference=w290) -> (reference out=w288:refnum<vi>, error out=w285:errorcluster, "Value"=w289:sgl)  [unwired: 1 in]
        n190 = call "input.vi"("位数(2)"=w284, "in"=w289) -> ("out"=w287:dbl, "值改变?"=w286:bool)
        n191 = property class="DigNum (严格)"(reference=w288, error in=w285, "Value"=w287) -> ()  [unwired: 2 out]
      }
      event "1#拨钮上下-上限", "1#拨钮下上-上限", "1#拨钮右左-上限", "1#拨钮左右-上限": Mouse Up {
        n192 = event-data() -> ("CtlRef"=w297:refnum<vi>)  [unwired: 1 in]
        n193 = property class="DigNum (严格)"(reference=w297) -> (reference out=w295:refnum<vi>, error out=w291:errorcluster, "Value"=w296:sgl)  [unwired: 1 in]
        n194 = call "input.vi"("位数(2)"=w293, "in"=w296) -> ("out"=w294:dbl, "值改变?"=w292:bool)
        n195 = property class="DigNum (严格)"(reference=w295, error in=w291, "Value"=w294) -> ()  [unwired: 2 out]
      }
      event "1#拨钮左右-锁上限", "1#拨钮右左-锁上限": Mouse Up {
        n196 = event-data() -> ("CtlRef"=w304:refnum<vi>)  [unwired: 1 in]
        n197 = property class="DigNum (严格)"(reference=w304) -> (reference out=w302:refnum<vi>, error out=w298:errorcluster, "Value"=w303:sgl)  [unwired: 1 in]
        n198 = call "input.vi"("位数(2)"=w300, "in"=w303) -> ("out"=w301:dbl, "值改变?"=w299:bool)
        n199 = property class="DigNum (严格)"(reference=w302, error in=w298, "Value"=w301) -> ()  [unwired: 2 out]
      }
      event "1#拨钮上下-下限", "1#拨钮下上-下限", "1#拨钮右左-下限", "1#拨钮左右-下限": Mouse Up {
        n200 = event-data() -> ("CtlRef"=w311:refnum<vi>)  [unwired: 1 in]
        n201 = property class="DigNum (严格)"(reference=w311) -> (reference out=w309:refnum<vi>, error out=w305:errorcluster, "Value"=w310:sgl)  [unwired: 1 in]
        n202 = call "input.vi"("位数(2)"=w307, "in"=w310) -> ("out"=w308:dbl, "值改变?"=w306:bool)
        n203 = property class="DigNum (严格)"(reference=w309, error in=w305, "Value"=w308) -> ()  [unwired: 2 out]
      }
      event "1#拨钮左右-锁下限", "1#拨钮右左-锁下限": Mouse Up {
        n204 = event-data() -> ("CtlRef"=w318:refnum<vi>)  [unwired: 1 in]
        n205 = property class="DigNum (严格)"(reference=w318) -> (reference out=w316:refnum<vi>, error out=w312:errorcluster, "Value"=w317:sgl)  [unwired: 1 in]
        n206 = call "input.vi"("位数(2)"=w314, "in"=w317) -> ("out"=w315:dbl, "值改变?"=w313:bool)
        n207 = property class="DigNum (严格)"(reference=w316, error in=w312, "Value"=w315) -> ()  [unwired: 2 out]
      }
      event "1#拨钮左右-上参考", "1#拨钮右左上参考", "1#拨钮下上-上参考", "1#拨钮上下-上参考": Mouse Up {
        n208 = event-data() -> ("CtlRef"=w325:refnum<vi>)  [unwired: 1 in]
        n209 = property class="DigNum (严格)"(reference=w325) -> (reference out=w323:refnum<vi>, error out=w319:errorcluster, "Value"=w324:sgl)  [unwired: 1 in]
        n210 = call "input.vi"("位数(2)"=w321, "in"=w324) -> ("out"=w322:dbl, "值改变?"=w320:bool)
        n211 = property class="DigNum (严格)"(reference=w323, error in=w319, "Value"=w322) -> ()  [unwired: 2 out]
      }
      event "1#拨钮左右-下参考", "1#拨钮右左-下参考", "1#拨钮下上-下参考", "1#拨钮上下-下参考": Mouse Up {
        n212 = event-data() -> ("CtlRef"=w332:refnum<vi>)  [unwired: 1 in]
        n213 = property class="DigNum (严格)"(reference=w332) -> (reference out=w330:refnum<vi>, error out=w326:errorcluster, "Value"=w331:sgl)  [unwired: 1 in]
        n214 = call "input.vi"("位数(2)"=w328, "in"=w331) -> ("out"=w329:dbl, "值改变?"=w327:bool)
        n215 = property class="DigNum (严格)"(reference=w330, error in=w326, "Value"=w329) -> ()  [unwired: 2 out]
      }
      event "1#拨钮左右-基准", "1#拨钮右左-基准", "1#拨钮下上-基准", "1#拨钮上下-基准": Mouse Up {
        n216 = event-data() -> ("CtlRef"=w339:refnum<vi>)  [unwired: 1 in]
        n217 = property class="DigNum (严格)"(reference=w339) -> (reference out=w337:refnum<vi>, error out=w333:errorcluster, "Value"=w338:sgl)  [unwired: 1 in]
        n218 = call "input.vi"("位数(2)"=w335, "in"=w338) -> ("out"=w336:dbl, "值改变?"=w334:bool)
        n219 = property class="DigNum (严格)"(reference=w337, error in=w333, "Value"=w336) -> ()  [unwired: 2 out]
      }
      event "1#拨钮右左-起点", "1#拨钮左右-起点", "1#拨钮上下-起点", "1#拨钮下上-起点": Mouse Up {
        n220 = event-data() -> ("CtlRef"=w346:refnum<vi>)  [unwired: 1 in]
        n221 = property class="DigNum (严格)"(reference=w346) -> (reference out=w344:refnum<vi>, error out=w340:errorcluster, "Value"=w345:dbl)  [unwired: 1 in]
        n222 = call "input.vi"("位数(2)"=w342, "in"=w345) -> ("out"=w343:dbl, "值改变?"=w341:bool)
        n223 = property class="DigNum (严格)"(reference=w344, error in=w340, "Value"=w343) -> ()  [unwired: 2 out]
      }
      event "1#拨钮左右-锁起点", "1#拨钮右左-锁起点": Mouse Up {
        n224 = event-data() -> ("CtlRef"=w353:refnum<vi>)  [unwired: 1 in]
        n225 = property class="DigNum (严格)"(reference=w353) -> (reference out=w351:refnum<vi>, error out=w347:errorcluster, "Value"=w352:dbl)  [unwired: 1 in]
        n226 = call "input.vi"("位数(2)"=w349, "in"=w352) -> ("out"=w350:dbl, "值改变?"=w348:bool)
        n227 = property class="DigNum (严格)"(reference=w351, error in=w347, "Value"=w350) -> ()  [unwired: 2 out]
      }
      event "1#拨钮左右-终点", "1#拨钮右左-终点", "1#拨钮下上-终点", "1#拨钮上下-终点": Mouse Up {
        n228 = event-data() -> ("CtlRef"=w360:refnum<vi>)  [unwired: 1 in]
        n229 = property class="DigNum (严格)"(reference=w360) -> (reference out=w358:refnum<vi>, error out=w354:errorcluster, "Value"=w359:dbl)  [unwired: 1 in]
        n230 = call "input.vi"("位数(2)"=w356, "in"=w359) -> ("out"=w357:dbl, "值改变?"=w355:bool)
        n231 = property class="DigNum (严格)"(reference=w358, error in=w354, "Value"=w357) -> ()  [unwired: 2 out]
      }
      event "1#拨钮左右-锁终点", "1#拨钮右左-锁终点": Mouse Up {
        n232 = event-data() -> ("CtlRef"=w367:refnum<vi>)  [unwired: 1 in]
        n233 = property class="DigNum (严格)"(reference=w367) -> (reference out=w365:refnum<vi>, error out=w361:errorcluster, "Value"=w366:dbl)  [unwired: 1 in]
        n234 = call "input.vi"("位数(2)"=w363, "in"=w366) -> ("out"=w364:dbl, "值改变?"=w362:bool)
        n235 = property class="DigNum (严格)"(reference=w365, error in=w361, "Value"=w364) -> ()  [unwired: 2 out]
      }
      event "1#拨钮上下-Y轴上限", "1#拨钮下上-Y轴上限", "1#拨钮右左-Y轴上限", "1#拨钮左右-Y轴上限": Mouse Up {
        n236 = event-data() -> ("CtlRef"=w374:refnum<vi>)  [unwired: 1 in]
        n237 = property class="DigNum (严格)"(reference=w374) -> (reference out=w372:refnum<vi>, error out=w368:errorcluster, "Value"=w373:dbl)  [unwired: 1 in]
        n238 = call "input.vi"("位数(2)"=w369, "in"=w373) -> ("out"=w371:dbl, "值改变?"=w370:bool)
        n239 = property class="DigNum (严格)"(reference=w372, error in=w368, "Value"=w371) -> ()  [unwired: 2 out]
      }
      event "1#拨钮上下-Y轴下限", "1#拨钮下上-Y轴下限", "1#拨钮右左-Y轴下限", "1#拨钮左右-Y轴下限": Mouse Up {
        n240 = event-data() -> ("CtlRef"=w381:refnum<vi>)  [unwired: 1 in]
        n241 = property class="DigNum (严格)"(reference=w381) -> (reference out=w379:refnum<vi>, error out=w375:errorcluster, "Value"=w380:dbl)  [unwired: 1 in]
        n242 = call "input.vi"("位数(2)"=w376, "in"=w380) -> ("out"=w378:dbl, "值改变?"=w377:bool)
        n243 = property class="DigNum (严格)"(reference=w379, error in=w375, "Value"=w378) -> ()  [unwired: 2 out]
      }
      event "1#拨钮上下-曲线点数", "1#拨钮下上-曲线点数", "1#拨钮右左-曲线点数", "1#拨钮左右-曲线点数": Mouse Up {
        n244 = event-data() -> ("CtlRef"=w388:refnum<vi>)  [unwired: 1 in]
        n245 = property class="DigNum (严格)"(reference=w388) -> (reference out=w386:refnum<vi>, error out=w382:errorcluster, "Value"=w387:dbl)  [unwired: 1 in]
        n246 = call "input.vi"("位数(2)"=0, "in"=w387) -> ("out"=w385:dbl, "值改变?"=w384:bool)
        n247 = property class="DigNum (严格)"(reference=w386, error in=w382, "Value"=w385) -> ()  [unwired: 2 out]
      }
    }
    "有值改变" <- w116
    n248 = global read "全局 1.vi" "PLC结果"() -> (→"PLC结果":T1)
    n249 = global read "全局 1.vi" "检测步骤"() -> (→"检测步骤":T2)
    n250 = global read "全局 1.vi" "PLC状态"() -> (→"PLC状态":T3)
    n251 = global read "全局SQL.vi" "cInvCode"() -> (→"物料编号":string)
    n252 = global read "全局 1.vi" "产线编号"() -> (→"产线编号":string)
    n253 = global read "全局 1.vi" "机台编号"() -> (→"机台编号":string)
    n254 = global read "全局 1.vi" "检测序号"() -> (→"检测序号":u16)
    n255 = property class="VI"("Front Panel.IsFrontmost"=TRUE ("前面板窗口:在最前")) -> ()  [unwired: 2 in, 2 out]
    n256 = global read "全局 1.vi" "力"() -> (→"力":sgl[])
    n257 = global read "全局 1.vi" "Exit"() -> (w118:bool)
    n258 = Or(x=w119, y=w118) -> (x .or. y?=w120:bool)
  }
  n259 = And(x=w4, y=TRUE) -> (x .and. y?=w5:bool)
  n260 = case shown="真" w5 {
    frame False {
    }
    frame True {
      n261 = invoke class="VI" method="FP.Close"() -> (reference out=w389:refnum<vi>, error out=w390:errorcluster)  [unwired: 3 in, 1 out]
      n262 = Close Reference(reference=w389, error in (no error)=w390) -> ()  [unwired: 1 out]
    }
  }
